vi "channel generation test.vi"() -> ()   [LabVIEW 2013, in "UI reference module tests.lvlib"]
uses:
  UI reference module tests.lvlib
  <vilib>/NI/Tag Bus/tag/tag descriptor.lvclass/tag descriptor.ctl
  <vilib>/NI/Tag Bus Module Framework/channel/TBM channel.lvclass/TBM channel.ctl
  <vilib>/NI/Tag Bus/tag/Data Type.ctl
  <vilib>/NI/Tag Bus Module Framework/channel/channel classification.ctl
  <vilib>/NI/Tag Bus/tag/read tag name.vi
  <vilib>/NI/Tag Bus/tag/read data type.vi
  <vilib>/NI/Tag Bus Module Framework/channel/Read channel classification.vi
  module/configuration/UI Reference configuration.lvclass
  <vilib>/NI/Tag Bus Module Framework/channel/TBM channel.lvclass
  <vilib>/NI/Tag Bus/tag/tag descriptor.lvclass
panel:
  out "pass":bool
  out "error out":errorcluster
  in  "App Refnum":refnum<vi>
  in  "Path":path
  in  "bool":bool
  in  "str":string
  out "i32 i":i32
  out "dbl i":dbl
  in  "i32":i32
  in  "dbl":dbl
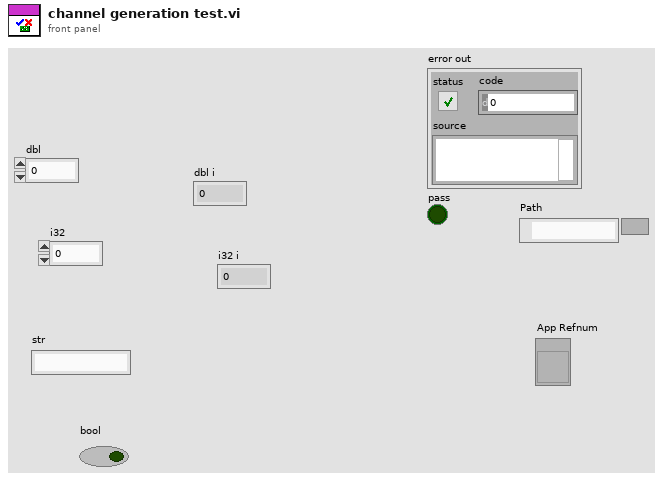
[diagram p1: front panel]
types:
  T1 = typedef "TBM channel.lvclass/channel classification.ctl" = enum16{"input data", "output data", "processing parameter", "processing result"}
  T2 = typedef "tag bus.lvlib/tag descriptor.lvclass/Data Type.ctl" = enum16{"Double", "Single", "I64", "I32", "I16", "I8", "U64", "U32", "U16", "U8", "Boolean", "String", "Array of Double", "Array of Single", "Array of I64", "Array of I32", "Array of I16", "Array of I8", "Array of U64", "Array of U32", "Array of U16", "Array of U8", "Array of Boolean", "Array of String"}
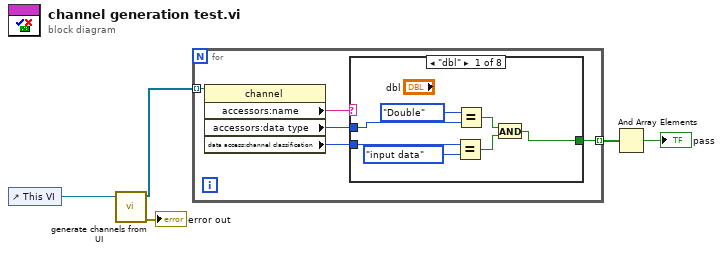
[diagram p0: block diagram]
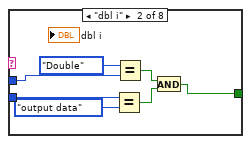
[diagram p2: hidden frame]
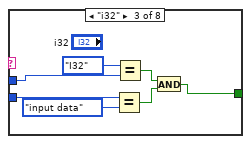
[diagram p3: hidden frame]
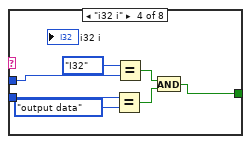
[diagram p4: hidden frame]
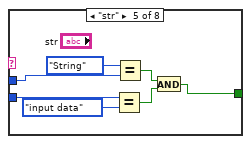
[diagram p5: hidden frame]
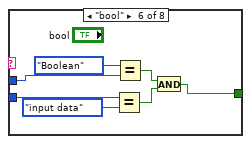
[diagram p6: hidden frame]
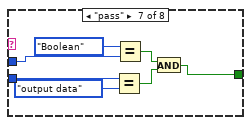
[diagram p7: hidden frame]
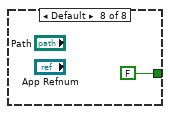
[diagram p8: hidden frame]
diagram:
  n1 = control-ref of="This VI"() -> (w5:refnum<vi>)
  n2 = call "generate channels from UI.vi"("VI Refnum"=w5) -> ("error out"=→"error out":errorcluster, "channels"=w3:refnum<class "TBM channel.lvclass">[])  [unwired: 9 in]
  n3 = for {
    tunnel: w3 -> [w10] mode=indexing
    tunnel: [w8] -> w2 mode=indexing
    n4 = property class="channel"(reference=w10) -> ("accessors:name"=w9:string, "accessors:data type"=w7:T2, "data access:channel classification"=w6:T1)  [unwired: 1 in, 2 out]
    n5 = case shown="\"dbl\"" w9 {
      tunnel: [w13 w20 w27 w34 w41 w48 w55 FALSE] -> w8
      tunnel: w7 -> [w16 w23 w30 w37 w44 w51 w58 _]
      tunnel: w6 -> [w17 w24 w31 w38 w45 w52 w59 _]
      frame "dbl" {
        n6 = Equal?(x=w17, y=channel_classification."input data") -> (x = y?=w15:bool)
        n7 = Equal?(x=Data_Type."Double", y=w16) -> (x = y?=w14:bool)
        n8 = And(x=w14, y=w15) -> (x .and. y?=w13:bool)
      }
      frame "dbl i" {
        n9 = Equal?(x=w24, y=channel_classification."output data") -> (x = y?=w22:bool)
        n10 = Equal?(x=Data_Type."Double", y=w23) -> (x = y?=w21:bool)
        n11 = And(x=w21, y=w22) -> (x .and. y?=w20:bool)
      }
      frame "i32" {
        n12 = Equal?(x=w31, y=channel_classification."input data") -> (x = y?=w29:bool)
        n13 = Equal?(x=Data_Type."I32", y=w30) -> (x = y?=w28:bool)
        n14 = And(x=w28, y=w29) -> (x .and. y?=w27:bool)
      }
      frame "i32 i" {
        n15 = Equal?(x=w38, y=channel_classification."output data") -> (x = y?=w36:bool)
        n16 = Equal?(x=Data_Type."I32", y=w37) -> (x = y?=w35:bool)
        n17 = And(x=w35, y=w36) -> (x .and. y?=w34:bool)
      }
      frame "str" {
        n18 = Equal?(x=w45, y=channel_classification."input data") -> (x = y?=w43:bool)
        n19 = Equal?(x=Data_Type."String", y=w44) -> (x = y?=w42:bool)
        n20 = And(x=w42, y=w43) -> (x .and. y?=w41:bool)
      }
      frame "bool" {
        n21 = Equal?(x=w52, y=channel_classification."input data") -> (x = y?=w50:bool)
        n22 = Equal?(x=Data_Type."Boolean", y=w51) -> (x = y?=w49:bool)
        n23 = And(x=w49, y=w50) -> (x .and. y?=w48:bool)
      }
      frame "pass" {
        n24 = Equal?(x=w59, y=channel_classification."output data") -> (x = y?=w57:bool)
        n25 = Equal?(x=Data_Type."Boolean", y=w58) -> (x = y?=w56:bool)
        n26 = And(x=w56, y=w57) -> (x .and. y?=w55:bool)
      }
      frame Default {
      }
    }
  }
  n27 = And Array Elements(Boolean array=w2) -> (logical AND=→"pass":bool)
